vi "Vision Server.vi"(8 "error in":errorcluster, 11 "port":u16=8254) -> (0 "error out":errorcluster)   [LabVIEW 2016, in "Vision Server.lvclass"]
uses:
  Vision Server.lvclass
  typedef/Message Type.ctl
  Vision Server.lvclass/Vision Server.ctl
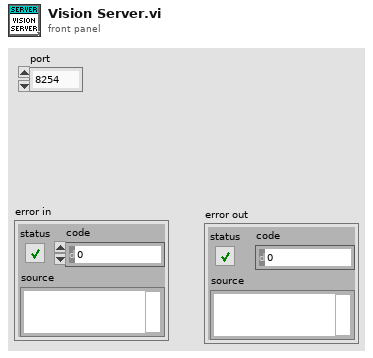
[diagram p1: front panel]
types:
  T1 = typedef "Vision Server.lvclass/Message Type.ctl" = cluster{"type":string, "message":string}
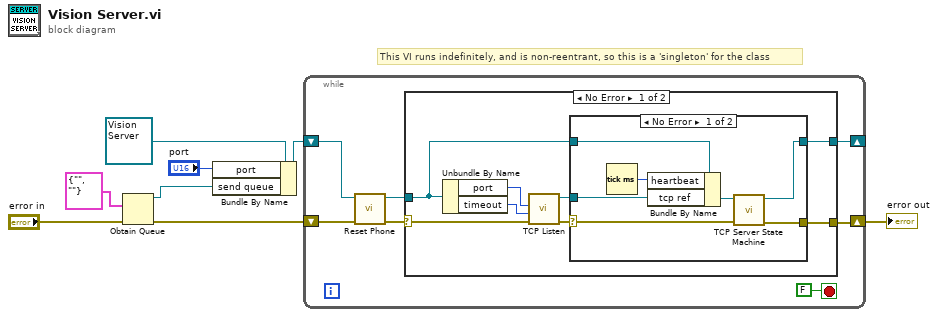
[diagram p0: block diagram]
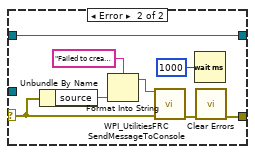
[diagram p2: hidden frame]
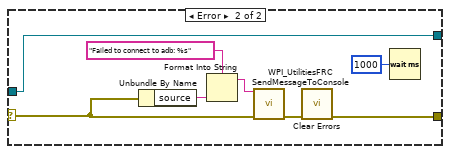
[diagram p3: hidden frame]
diagram:
  # "This VI runs indefinitely, and is non-reentrant, so this is a 'singleton' for the class"
  n1 = Obtain Queue(element data type=T1 {"type"="", "message"=""} ("Cluster"), error in (no error)="error in") -> (queue out=w4:refnum<queue>, error out=w2:errorcluster)  [unwired: 3 in, 1 out]
  n2 = Bundle By Name(cluster=refnum<class "Vision Server.lvclass"> refnum ("Vision Server.lvclass"), "port"="port", "send queue"=w4) -> (w1:refnum<class "Vision Server.lvclass">)
  n3 = while {
    shift-right: [w13] -> w8
    shift-left: w2 -> [w12]
    shift-right: [w14] -> _
    shift-left: w1 -> [w10]
    stop <- FALSE stop-if-true
    n4 = call "Reset Phone.vi"("error in (no error)"=w12, "Vision Server in"=w10) -> ("error out"=w11:errorcluster, "Vision Server out"=w9:refnum<class "Vision Server.lvclass">)  [unwired: 8 in]
    n5 = case shown="No Error" w11 {
      selector: w11 -> [w18 w40]
      tunnel: [w20 w46] -> w14
      tunnel: [w19 w39] -> w13
      tunnel: w9 -> [w17 w46]
      frame No Error {
        n6 = Unbundle By Name(w17) -> ("port"=w22:u16, "timeout"=w16:i32)
        n7 = call <vilib>:"TCP Listen.vi"("error in (no error)"=w18, "timeout ms (wait forever: -1)"=w16, "port"=w22) -> ("error out"=w23:errorcluster, "connection ID"=w21:refnum<k5>)  [unwired: 4 in, 3 out]
        n8 = case shown="No Error" w23 {
          selector: w23 -> [w30 w31]
          tunnel: [w29 w32] -> w19
          tunnel: [w28 w38] -> w20
          tunnel: w17 -> [w27 w38]
          tunnel: w21 -> [w25 _]
          frame No Error {
            n9 = Tick Count (ms)() -> (millisecond timer value=w24:u32)
            n10 = Bundle By Name(cluster=w27, "heartbeat"=w24, "tcp ref"=w25) -> (w26:refnum<class "Vision Server.lvclass">)
            n11 = call "TCP Server State Machine.vi"("error in"=w30, "Vision Server in"=w26) -> ("error out"=w29:errorcluster, "Vision Server out"=w28:refnum<class "Vision Server.lvclass">)  [unwired: 8 in]
          }
          frame Error {
            n12 = Unbundle By Name(w31) -> ("source"=w35:string)
            n13 = Format Into String(format string="Failed to create server: %s", w35) -> (resulting string=w33:string)  [unwired: 2 in, 1 out]
            n14 = call <vilib>:"WPI_UtilitiesFRC SendMessageToConsole.vi"("Message"=w33, "error in (no error)"=w31) -> ("error out"=w36:errorcluster)  [unwired: 13 in]
            n15 = Wait (ms)(milliseconds to wait=u32 1000) -> ()  [unwired: 1 out]
            n16 = call <vilib>:"Clear Errors.vi"("error in (no error)"=w36) -> ("error out"=w32:errorcluster)  [unwired: 5 in, 1 out]
          }
        }
      }
      frame Error {
        n17 = Unbundle By Name(w40) -> ("source"=w44:string)
        n18 = Format Into String(format string="Failed to connect to adb: %s", w44) -> (resulting string=w42:string)  [unwired: 2 in, 1 out]
        n19 = call <vilib>:"WPI_UtilitiesFRC SendMessageToConsole.vi"("Message"=w42, "error in (no error)"=w40) -> ("error out"=w41:errorcluster)  [unwired: 13 in]
        n20 = call <vilib>:"Clear Errors.vi"("error in (no error)"=w41) -> ("error out"=w39:errorcluster)  [unwired: 5 in, 1 out]
        n21 = Wait (ms)(milliseconds to wait=u32 1000) -> ()  [unwired: 1 out]
      }
    }
  }
  "error out" <- w8
